vi "temp_sensor_project.vi"() -> ()   [LabVIEW 2019]
uses:
  <vilib>/Instr/_visa.llb/VISA Configure Serial Port (Instr).vi
panel:
  in  "Millisecond timer value":u32
  out "Table":string[][](table)
  in  "stop":bool
  in  "VISA resource name":refnum<visa-resource-name>
  in  "Write to file":bool
  out "?":bool
  in  "Path":path
  out "Waveform Chart":dbl[](graph)
  out "Thermometer, °C":dbl(slide) scale=-55.0..125.0 scale format="%#.2g"
  in  "High temperature level":dbl(slide) scale=-55.0..125.0
  in  "Low temperature level":dbl(slide) scale=-55.0..125.0
  out ">High":bool
  out "Normal":bool
  out "<Low":bool
  # "Device control"
  # "Temperature level parameters"
  # "Current temperature level data"
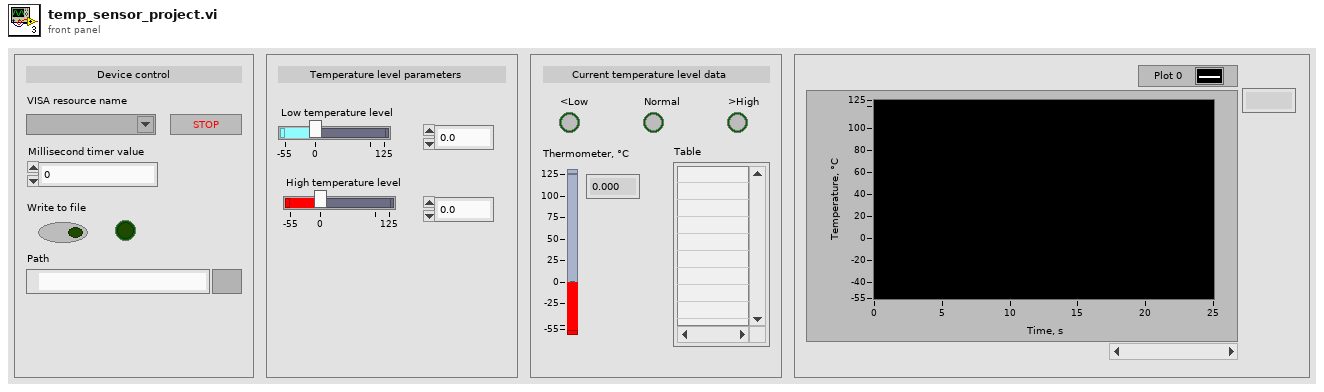
[diagram p1: front panel]
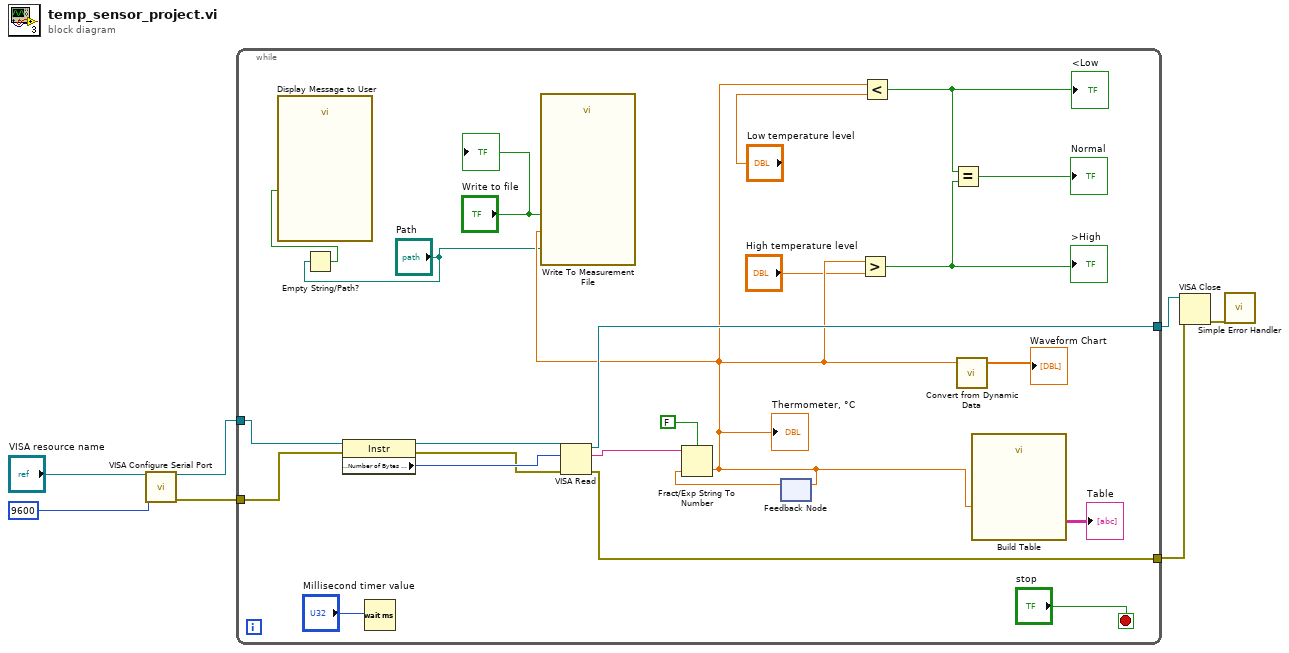
[diagram p0: block diagram]
diagram:
  n1 = call-poly "VISA Configure Serial Port"("VISA resource name"="VISA resource name", "baud rate (9600)"=u32 9600) -> ("VISA resource name out"=w5:refnum<visa-resource-name>, "error out"=w4:errorcluster)  [unwired: 12 in]
  n2 = while {
    tunnel: w5 -> [w18]
    tunnel: w4 -> [w17]
    tunnel: [w24] -> w3
    tunnel: [w23] -> w1
    stop <- "stop" stop-if-true
    n3 = Empty String/Path?(string/path="Path") -> (empty?=w8:bool)
    n4 = call "Display Message to User"("Enable"=w8) -> ()  [unwired: 9 in, 2 out]
    n5 = property class="Instr"(reference=w18, error in=w17) -> (reference out=w29:refnum<visa-resource-name>, error out=w27:errorcluster, "Serial Settings:Number of Bytes at Serial Port"=w28:u32)
    n6 = Wait (ms)(milliseconds to wait="Millisecond timer value") -> ()  [unwired: 1 out]
    n7 = VISA Read(VISA resource name=w29, byte count=w28, error in (no error)=w27) -> (VISA resource name out=w24:refnum<visa-resource-name>, read buffer=w26:string, error out=w23:errorcluster)  [unwired: 1 out]
    n8 = feedback #1() -> (w21:dbl)  [unwired: 1 in]
    n9 = Fract/Exp String To Number(use system decimal point (T)=FALSE, string=w26, default (0 dbl)=w21) -> (number=w14:dbl)  [unwired: 1 in, 1 out]
    "Thermometer, °C" <- w14
    n10 = call "Write To Measurement File"("Signals"=w14, "Enable"="Write to file", "Filename"="Path") -> ()  [unwired: 14 in, 3 out]
    n11 = feedback-in #1(w14) -> ()
    n12 = Greater?(x=w14, y="High temperature level") -> (0:w11:bool)
    ">High" <- w11
    n13 = Less?(x=w14, y="Low temperature level") -> (x < y?=w12:bool)
    "<Low" <- w12
    n14 = Equal?(x=w12, y=w11) -> (x = y?=→"Normal":bool)
    n15 = call "Convert from Dynamic Data"("Dynamic Data Type"=w14) -> ("Array"=→"Waveform Chart":dbl[])  [unwired: 3 in]
    n16 = call "Build Table"("Signals"=w14) -> ("Table"=→"Table":string[][])  [unwired: 4 in, 6 out]
    "?" <- "Write to file"
  }
  n17 = VISA Close(VISA resource name=w3, error in (no error)=w1) -> (error out=w2:errorcluster)
  n18 = call <vilib>:"Simple Error Handler.vi"("error in (no error)"=w2) -> ()  [unwired: 4 in, 5 out]
